vi "hello world.vi"() -> ()   [LabVIEW 2023]
panel:
  in  "Tab Control":enum32{"Page 1", "Page 2"}(tab)
  in  "bool 3":bool
  in  "stop 2":bool
  in  "Boolean":bool
  out "Boolean 2":bool
  in  "stop":bool
  out "Numeric":i32
  in  "VISA resource name":refnum<visa-resource-name>
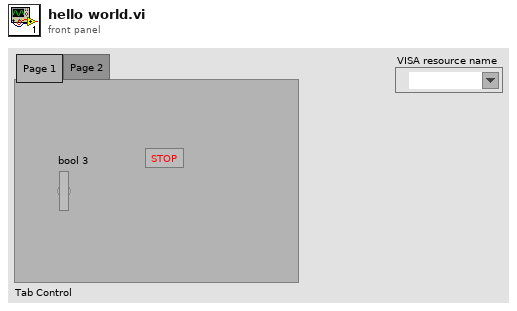
[diagram p1: front panel]
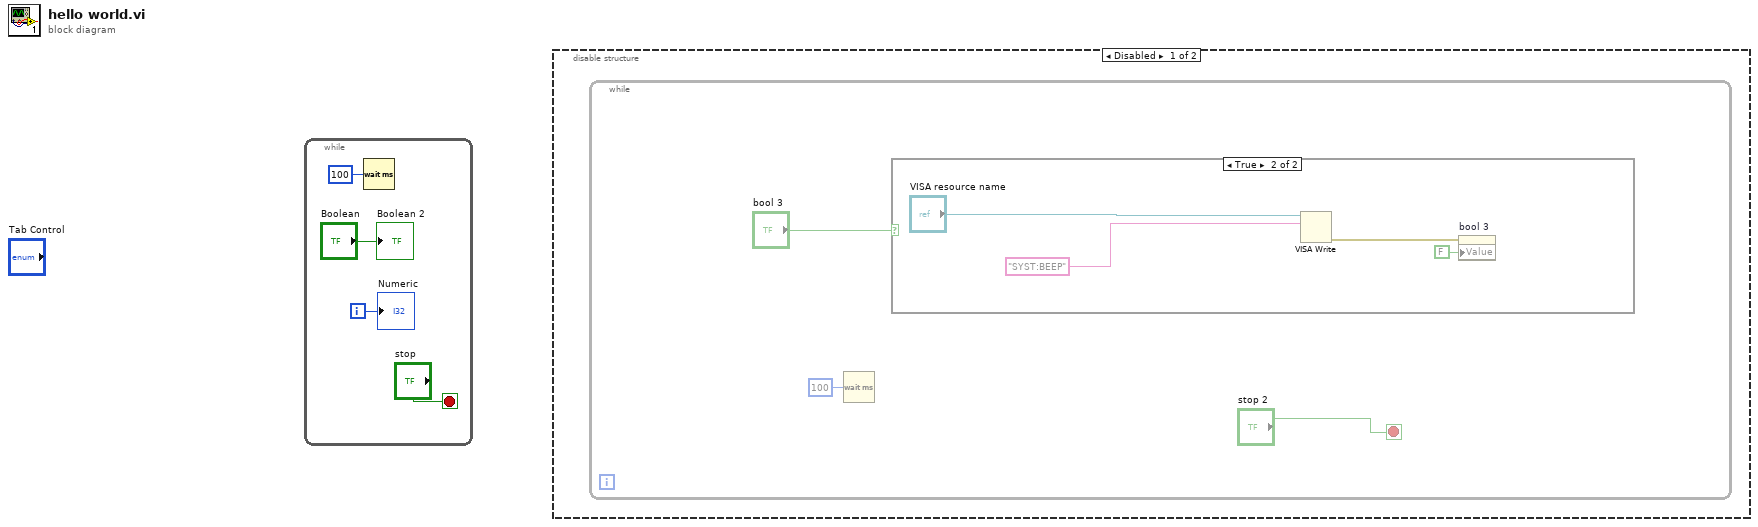
[diagram p0: block diagram]
diagram:
  n1 = while {
    i -> [w2]
    stop <- "stop" stop-if-true
    n2 = Wait (ms)(milliseconds to wait=100) -> ()  [unwired: 1 out]
    "Boolean 2" <- "Boolean"
    "Numeric" <- w2
  }
  n3 = disable-structure shown="Disabled" {
    frame Disabled {
      n4 = while {
        stop <- "stop 2" stop-if-true
        n5 = Wait (ms)(milliseconds to wait=100) -> ()  [unwired: 1 out]
        n6 = case shown="True" "bool 3" {
          frame False {
          }
          frame True {
            n7 = VISA Write(VISA resource name="VISA resource name", write buffer="SYST:BEEP") -> (error out=w8:errorcluster)  [unwired: 1 in, 2 out]
            n8 = property on="bool 3" class="Bool (strict)"(error in=w8, "Value"=FALSE ("Boolean 3")) -> ()  [unwired: 1 in, 2 out]
          }
        }
      }
    }
    frame Enabled {
    }
  }
